vi "Kettle Temperature.vi"(1 "Outside Temp":dbl, 2 "Buffer(iteration)":u32, 3 "Buffer(Kettle Temp.)":dbl=25.0, 4 "Kettle Condition":bool) -> (0 "Kettle Temp.":dbl)   [LabVIEW 2020]
panel:
  out "error out":errorcluster
  # "This is the subVI of \"Ketlte.vi\". Please have look at master VI\nfor more information."
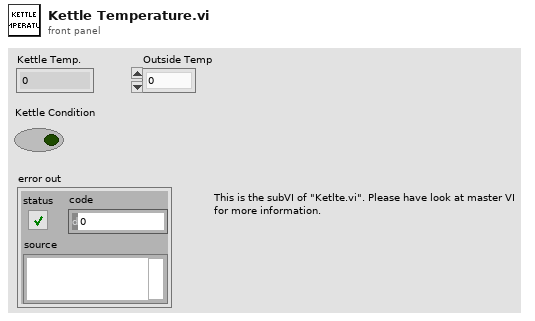
[diagram p1: front panel]
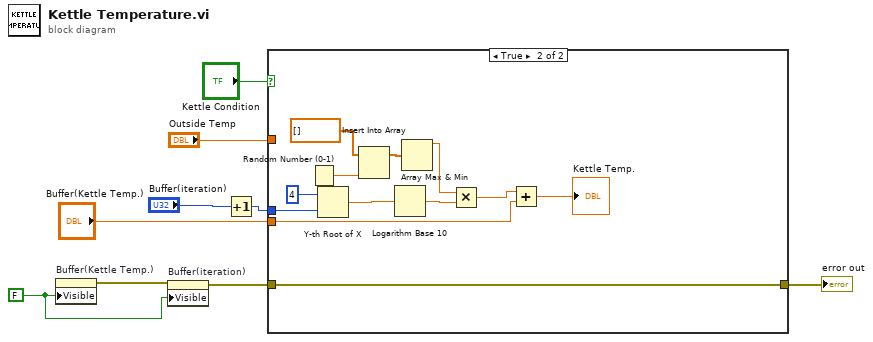
[diagram p0: block diagram]
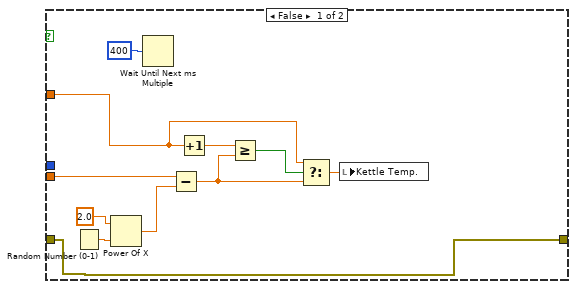
[diagram p2: hidden frame]
diagram:
  w6 = FALSE ("Visible")
  n1 = property on="Buffer(Kettle Temp.)" class="DigNum (strict)"("Visible"=w6) -> (error out=w4:errorcluster)  [unwired: 2 in, 1 out]
  n2 = property on="Buffer(iteration)" class="DigNum (strict)"(error in=w4, "Visible"=w6) -> (error out=w3:errorcluster)  [unwired: 1 in, 1 out]
  n3 = Increment(x="Buffer(iteration)") -> (x+1=w8:u32)
  n4 = case shown="True" "Kettle Condition" {
    tunnel: "Buffer(Kettle Temp.)" -> [w16 w22]
    tunnel: w8 -> [_ w28]
    tunnel: [w11 w24] -> w2
    tunnel: w3 -> [w11 w24]
    tunnel: "Outside Temp" -> [w10 _]
    frame False {
      n5 = Random Number (0-1)() -> (number: 0 to 1=w18:dbl)
      n6 = Power Of X(1:w18, 2:2.0 ("y")) -> (0:w19:dbl)
      n7 = Wait Until Next ms Multiple(millisecond multiple=u32 400) -> ()  [unwired: 1 out]
      n8 = Subtract(x=w16, y=w19) -> (x-y=w13:dbl)
      n9 = Increment(x=w10) -> (x+1=w14:dbl)
      n10 = Greater Or Equal?(x=w14, y=w13) -> (x >= y?=w12:bool)
      n11 = Select(t=w10, s=w12, f=w13) -> (s? t:f=w15:dbl)
      n12 = local write "Kettle Temp."(w15) -> ()
    }
    frame True {
      n13 = Random Number (0-1)() -> (number: 0 to 1=w32:dbl)
      n14 = Y-th Root of X(1:w28, 2:4 ("y")) -> (0:w27:dbl)
      n15 = Insert Into Array(array=dbl[] [] ("Array"), new element=w32) -> (w30:dbl[])  [unwired: 1 in]
      n16 = Logarithm Base 10(1:w27) -> (0:w31:dbl)
      n17 = Array Max & Min(array=w30) -> (max value=w29:dbl)  [unwired: 3 out]
      n18 = Multiply(x=w29, y=w31) -> (x*y=w23:dbl)
      n19 = Add(x=w23, y=w22) -> (x+y=→"Kettle Temp.":dbl)
    }
  }
  "error out" <- w2
